vi "EnqueueMessage(MsgObj).vi"(5 "In Front? (F)":bool, 7 "Timeout (-1 ms)":i32, 8 "error in (no error)":errorcluster, 10 "Message":refnum<class "Message.lvclass">, 11 "MessageQueue":refnum<class "MessageQueue.lvclass">) -> (0 "error out":errorcluster, 3 "MessageQueue out":refnum<class "MessageQueue.lvclass">, 4 "Timed Out?":bool)   [LabVIEW 2009, in "LapDog.Messaging.v2.lvlib" / "MessageQueue.lvclass"]
doc: "Adds a message object to the queue. By default the message is added to the rear of the queue. Set 'In Front?' to TRUE to add the message to the front of the queue.\n\nThis method executes regardless of the error in state."
uses:
  MessageQueue.lvclass
  MessageObject/Message.lvclass
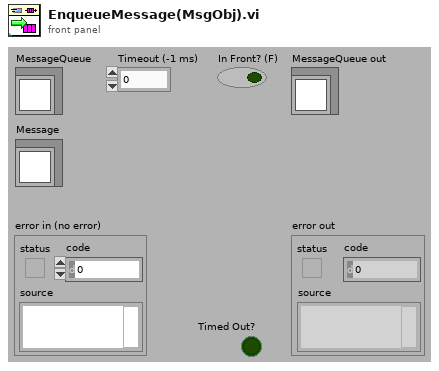
[diagram p1: front panel]
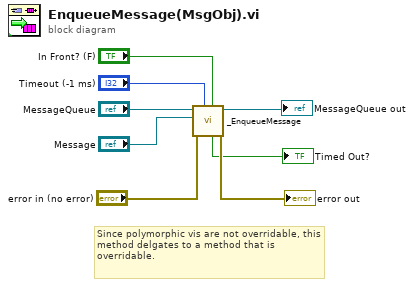
[diagram p0: block diagram]
diagram:
  # "Since polymorphic vis are not overridable, this method delgates to a method that is overridable."
  n1 = call-dynamic "_EnqueueMessage.vi"("In Front? (F)"="In Front? (F)", "Timeout (-1 ms)"="Timeout (-1 ms)", "error in (no error)"="error in (no error)", "Message"="Message", "MessageQueue"="MessageQueue") -> ("error out"=→"error out":errorcluster, "MessageQueue out"=→"MessageQueue out":refnum<class "MessageQueue.lvclass">, "Timed Out?"=→"Timed Out?":bool)  [unwired: 4 in]
